vi "Get SA Frequency.vi"(8 "error in (no error)":errorcluster, 11 "SPECAN_IQSLOT in":refnum<class "SPECAN_IQSLOT.lvclass">) -> (0 "error out":errorcluster, 3 "SPECAN_IQSLOT out":refnum<class "SPECAN_IQSLOT.lvclass">)   [LabVIEW 2018, in "SPECAN_IQSLOT.lvlib" / "SPECAN_IQSLOT.lvclass"]
uses:
  SPECAN_IQSLOT.lvclass
  C:/Sequence Automation/Plugins/Measurement Interface.lvlibp/Measurement Interface.lvclass
  Plugins/Measurement Interface.lvlibp/Private Methods/Measurement Parameters/Read Measurement Parameters.vi
  Plugins/String Database.lvlibp/String Database.lvclass
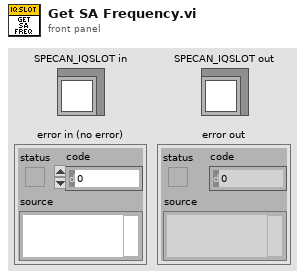
[diagram p1: front panel]
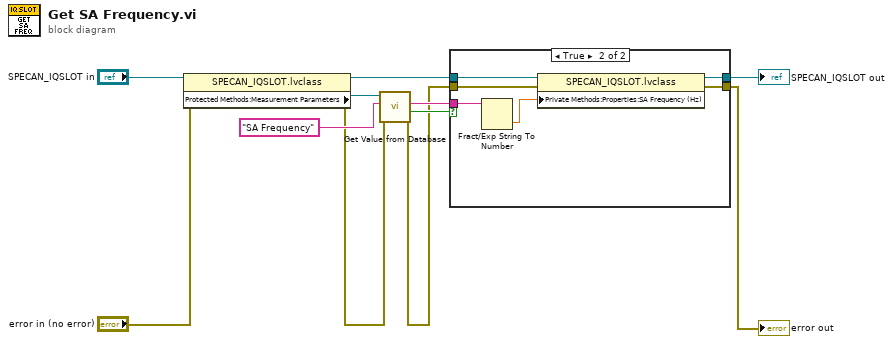
[diagram p0: block diagram]
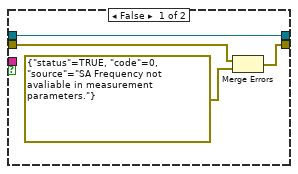
[diagram p2: hidden frame]
diagram:
  n1 = property class="SPECAN_IQSLOT.lvclass"(reference="SPECAN_IQSLOT in", error in="error in (no error)") -> (reference out=w5:refnum<class "SPECAN_IQSLOT.lvclass">, error out=w9:errorcluster, "Protected Methods:Measurement Parameters"=w11:refnum<class "String Database.lvclass">)
  n2 = call "Get Value from Database.vi"("error in (no error)"=w9, "Entry Name"="SA Frequency", "Message in"=w11) -> ("error out"=w3:errorcluster, "Entry Found"=w8:bool, "Entry Value"=w4:string)  [unwired: 5 in, 1 out]
  n3 = case shown="True" w8 {
    tunnel: w5 -> [w15 w21]
    tunnel: w4 -> [_ w16]
    tunnel: w3 -> [w13 w20]
    tunnel: [w15 w19] -> w2
    tunnel: [w12 w18] -> w1
    frame False {
      n4 = Merge Errors(w13, errorcluster {"status"=TRUE, "code"=0, "source"="SA Frequency not avaliable in measurement parameters."} ("error out")) -> (w12:errorcluster)
    }
    frame True {
      n5 = Fract/Exp String To Number(string=w16) -> (number=w17:dbl)  [unwired: 3 in, 1 out]
      n6 = property class="SPECAN_IQSLOT.lvclass"(reference=w21, error in=w20, "Private Methods:Properties:SA Frequency (Hz)"=w17) -> (reference out=w19:refnum<class "SPECAN_IQSLOT.lvclass">, error out=w18:errorcluster)
    }
  }
  "error out" <- w1
  "SPECAN_IQSLOT out" <- w2
